vi "_Create Data Queue.vi"(7 "max queue size (-1, unlimited)":i32=-1, 8 "error in (no error)":errorcluster, 9 "create if not found? (T)":bool=TRUE, 11 "Name":string) -> (0 "error out":errorcluster, 1 "created new?":bool, 3 "Queue out":refnum<queue>)   [LabVIEW 2014, in "JKI-State-Machine-Plus.lvlib"]
uses:
  JKI-State-Machine-Plus.lvlib
  _Cross JKI StateMachine State Data.ctl
  _JKISM_MSG_TYPE.ctl
  _Cross JKI StateMachine State Response.ctl
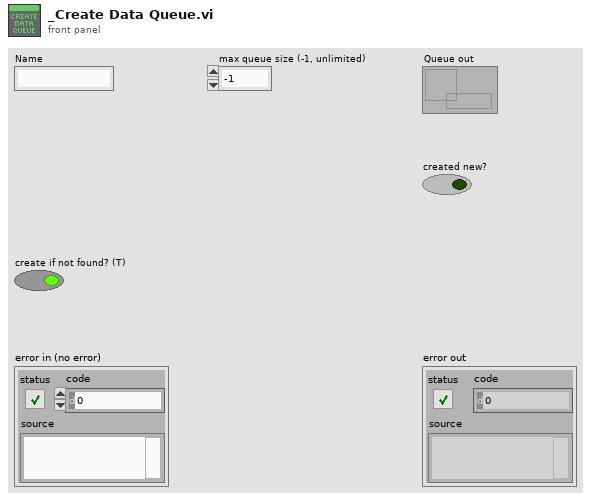
[diagram p1: front panel]
types:
  T1 = typedef "JKI-State-Machine-Plus.lvlib/_Cross JKI StateMachine State Data.ctl" = cluster{"Msg Type":T2, "state":string, "args":string, "source":string, "RespQ":refnum<queue>, "Pre-State":string, "Arg-State":string}
  T2 = typedef "JKI-State-Machine-Plus.lvlib/_JKISM_MSG_TYPE.ctl" = enum16{"Sync Message(@)", "Async Message(->)", "Broadcast Status(-><all>)", "Aync Response"}
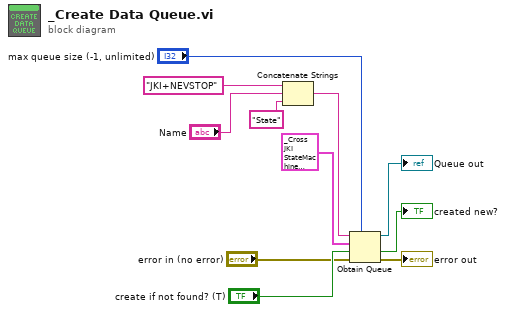
[diagram p0: block diagram]
diagram:
  n1 = Concatenate Strings("JKI+NEVSTOP" ("string"), "Name", "State" ("string in")) -> (w8:string)
  n2 = Obtain Queue(max queue size (-1, unlimited)="max queue size (-1, unlimited)", name (unnamed)=w8, element data type=T1 {"Msg Type"=enum."Sync Message(@)", "state"="", "args"="", "source"="", "RespQ"=refnum, "Pre-State"="", "Arg-State"=""} ("Cross JKI State Machine State"), create if not found? (T)="create if not found? (T)", error in (no error)="error in (no error)") -> (queue out=→"Queue out":refnum<queue>, created new?=→"created new?":bool, error out=→"error out":errorcluster)
